vi "Read View Channel info.vi"(8 "error in":errorcluster, 11 "channel in":refnum<class "Channel.lvclass">) -> (0 "error out":errorcluster, 2 "channel info":T1, 3 "channel out":refnum<class "Channel.lvclass">)   [LabVIEW 2015, in "Channel.lvclass"]
uses:
  Channel.lvclass
  ChannelDisplayInfo.ctl
  Channel.lvclass/Channel.ctl
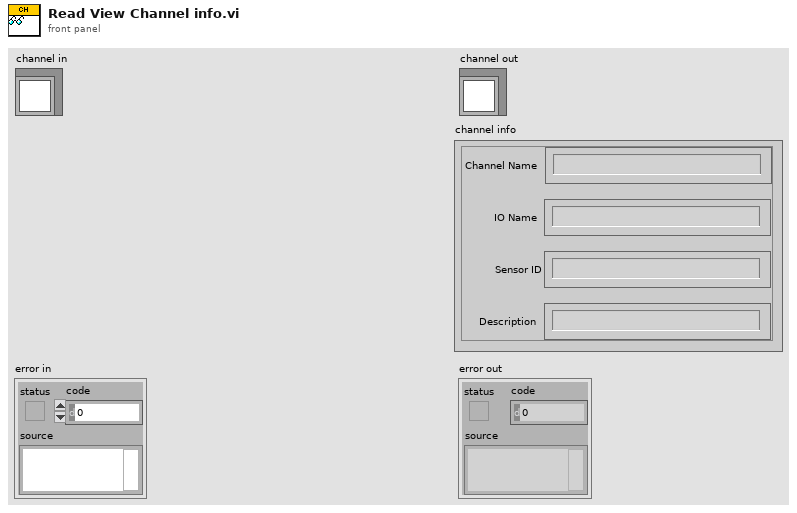
[diagram p1: front panel]
types:
  T1 = typedef "Channel.lvclass/ChannelDisplayInfo.ctl" = cluster{"IO Name":string, "Sensor ID":string, "Channel Name":string, "Description ":string}
  T2 = typedef "cRIORepo.lvclass/ChannelData.ctl" = cluster{"channel group":string, "channel name":string, "IO ":string, "sensor ID":string, "description":string, "system":string, "channel type":string}
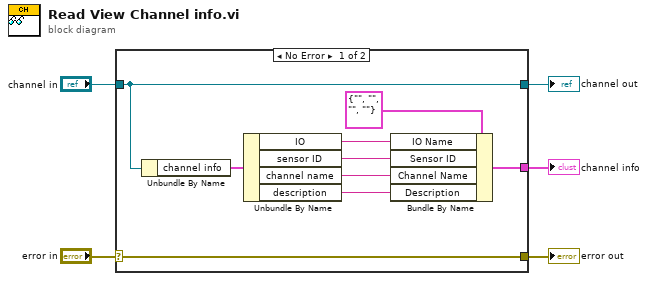
[diagram p0: block diagram]
diagram:
  n1 = case shown="No Error" "error in" {
    selector: "error in" -> [w14 w15]
    tunnel: [w14 w15] -> w4
    tunnel: [w13 w16] -> w2
    tunnel: "channel in" -> [w13 w16]
    tunnel: [w7 _] -> w1
    frame No Error {
      n2 = Unbundle By Name(w13) -> ("channel info"=w8:T2)
      n3 = Unbundle By Name(w8) -> ("IO"=w12:string, "sensor ID"=w11:string, "channel name"=w10:string, "description"=w9:string)
      n4 = Bundle By Name(cluster=T1 {"IO Name"="", "Sensor ID"="", "Channel Name"="", "Description "=""} ("channel info"), "IO Name"=w12, "Sensor ID"=w11, "Channel Name"=w10, "Description"=w9) -> (w7:T1)
    }
    frame Error {
    }
  }
  "error out" <- w4
  "channel out" <- w2
  "channel info" <- w1
